vi "Destroy Msg Queue__ogtk.vi"(4 "error in (no error)":errorcluster, 6 "Destroy Response Notifiers? (T)":bool, 7 "msg queue":T3) -> (0 "error out":errorcluster, 2 "massages":T1[](array[typedef]), 3 "queue name":string)   [LabVIEW 2009]
doc: "Destroys the specified message queue and returns any messages that are in the queue and optionally destroys all response notifiers. All Insert Msg Queue Element and Remove Msg Queue Element VIs that are currently waiting on this queue will time out immediately and return an error."
uses:
  Msg Queue RefNum__ogtk.ctl
  Msg Cluster__ogtk.ctl
panel:
  # "[OpenG VI Tags] ***Do Not Remove***"
  # "Destroy Msg Queue.vi\n\nDestroys the specified message queue and returns any messages that are in the qu\n\nPlease visit http://www.OpenG.org to learn about the\nOpen Source LabVIEW software movement.\n\nNOTICE -- YOU MUST LEAVE THIS NOTICE IN PLACE.  PER THE TERMS OF THE LICENSE BELOW, YOU MAY SUBLICENSE THIS SOFTWARE \nIN ANY WAY THAT DOES NOT CONFLICT WITH THIS LICENSE.\n\n### BSD License (http://www.opensource.org/licenses/bsd-license.php) Begin ###\n\nCopyright (c) 2002, Jim Kring <jim@jimkring.com>\n\nAll rights reserved.\n\nRedistribution and use in source and binary forms, with or without modification, are permitted provided that the following conditions are met:\n\n    * Redistributions of source code must retain the above copyright notice, this list of conditions and the following disclaimer.\n    * Redistributions in binary form must reproduce the above copyright notice, this list of conditions and the following disclaimer in the \n       documentation and/or other materials provided with the distribution.\n    * Neither the name of SciWare, James Kring, Inc., nor the names of its contributors may be used to endorse or promote products derived \n       from this software without specific prior written permission.\n\nTHIS SOFTWARE IS PROVIDED BY THE COPYRIGHT HOLDERS AND CONTRIBUTORS \"AS IS\" AND ANY EXPRESS OR IMPLIED WARRANTIES, \nINCLUDING, BUT NOT LIMITED TO, THE IMPLIED WARRANTIES OF MERCHANTABILITY AND FITNESS FOR A PARTICULAR PURPOSE ARE \nDISCLAIMED. IN NO EVENT SHALL THE COPYRIGHT OWNER OR CONTRIBUTORS BE LIABLE FOR ANY DIRECT, INDIRECT, INCIDENTAL,\n SPECIAL, EXEMPLARY, OR CONSEQUENTIAL DAMAGES (INCLUDING, BUT NOT LIMITED TO, PROCUREMENT OF SUBSTITUTE GOODS OR \nSERVICES; LOSS OF USE, DATA, OR PROFITS; OR BUSINESS INTERRUPTION) HOWEVER CAUSED AND ON ANY THEORY OF LIABILITY, \nWHETHER IN CONTRACT, STRICT LIABILITY, OR TORT (INCLUDING NEGLIGENCE OR OTHERWISE) ARISING IN ANY WAY OUT OF THE USE \nOF THIS SOFTWARE, EVEN IF ADVISED OF THE POSSIBILITY OF SUCH DAMAGE.\n\n### BSD License End ###"
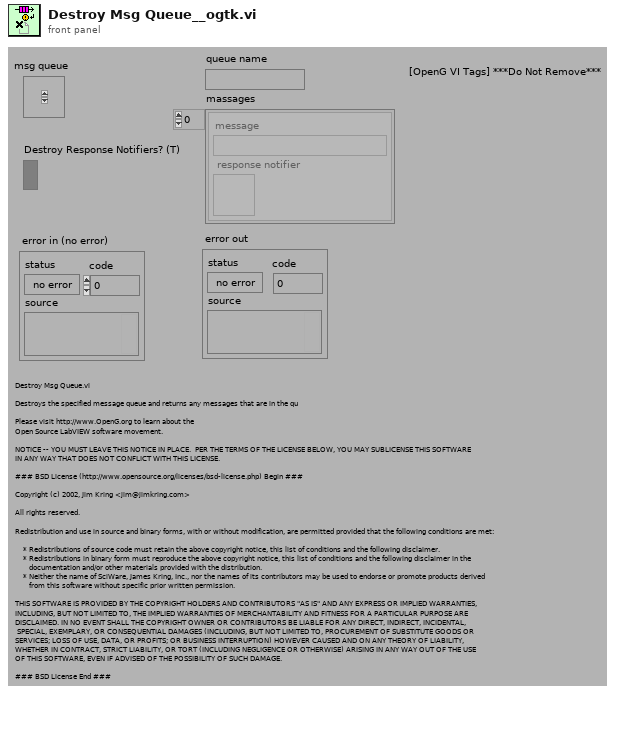
[diagram p1: front panel]
types:
  T1 = typedef "Msg Cluster__ogtk.ctl" = cluster{"message":string, "response notifier":T2}
  T2 = typedef "Notifier RefNum" = refnum<k1>
  T3 = typedef "Msg Queue RefNum__ogtk.ctl" = refnum<k1>
  T4 = typedef "Queue RefNum" = refnum<k1>
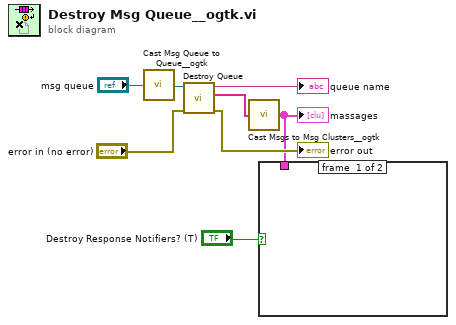
[diagram p0: block diagram]
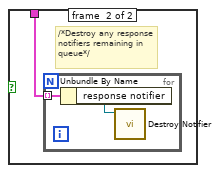
[diagram p2: hidden frame]
diagram:
  n1 = call "Cast Msg Queue to Queue__ogtk.vi"("msg queue"="msg queue") -> ("queue"=w5:T4)  [unwired: 4 in]
  n2 = call <vilib>:"Destroy Queue.vi"("error in (no error)"="error in (no error)", "queue"=w5) -> ("error out"=→"error out":errorcluster, "remaining elements"=w3:string[], "queue name"=→"queue name":string)  [unwired: 3 in]
  n3 = call "Cast Msgs to Msg Clusters__ogtk.vi"("queue elements"=w3) -> ("massages"=w2:T1[])  [unwired: 4 in]
  "massages" <- w2
  n4 = case shown="True" "Destroy Response Notifiers? (T)" {
    tunnel: w2 -> [_ w9]
    frame #0 {
    }
    frame #1 {
      # "/*Destroy any response notifiers remaining in queue*/"
      n5 = for {
        tunnel: w9 -> [w11] mode=indexing
        n6 = Unbundle By Name(w11) -> ("response notifier"=w10:T2)
        n7 = call <vilib>:"Destroy Notifier.vi"("notifier"=w10) -> ()  [unwired: 4 in, 3 out]
      }
    }
  }
